vi "RW_LiveVIew.vi"(9 "Task":enum16{"Read", "Write", "Init"}(ring), 11 "Plots":refnum<vi>[](array[refnum])) -> ()   [LabVIEW 2022 SP3]
uses:
  <vilib>/Utility/miscctls.llb/LVRangeTypeDef.ctl
panel:
  out "Data":T1[][](array[typedef])
  out "Pref Path":path
  out "File Out":string
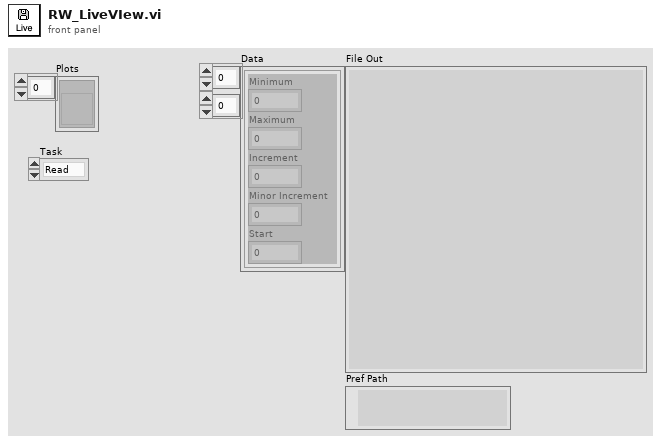
[diagram p1: front panel]
types:
  T1 = typedef "LVRangeTypeDef.ctl" = cluster{"Minimum":dbl, "Maximum":dbl, "Increment":dbl, "Minor Increment":dbl, "Start":dbl}
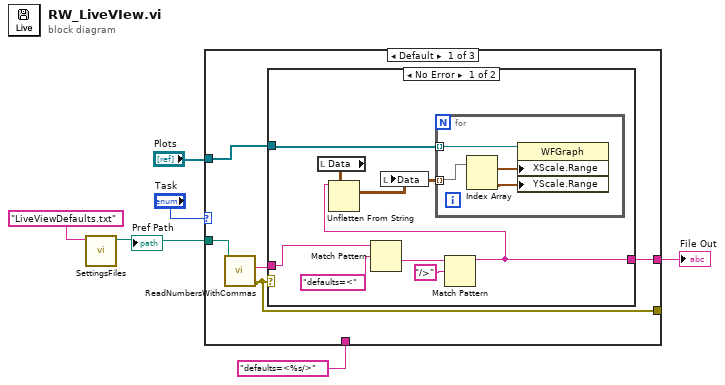
[diagram p0: block diagram]
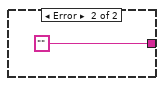
[diagram p2: hidden frame]
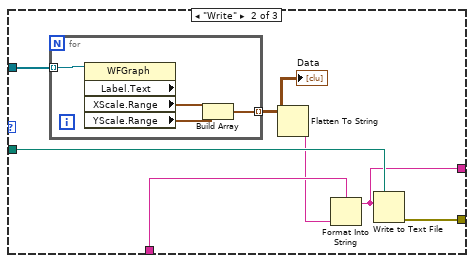
[diagram p3: hidden frame]
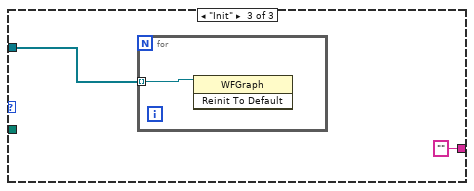
[diagram p4: hidden frame]
diagram:
  n1 = call "SettingsFiles.vi"("settings file name"="LiveViewDefaults.txt" ("name or relative path")) -> ("file path"=w1:path)  [unwired: 9 in, 1 out]
  "Pref Path" <- w1
  n2 = case shown="Default" "Task" {
    tunnel: w1 -> [w11 w31 _]
    tunnel: [w9 w30 _] -> _
    tunnel: [w8 w25 "" ("Notes")] -> w6
    tunnel: "defaults=<%s/>" ("format string") -> [_ w29 _]
    tunnel: "Plots" -> [w7 w28 w37]
    frame Default {
      n3 = call "ReadNumbersWithCommas.vi"("file (use dialog)"=w11) -> ("error out"=w9:errorcluster, "text"=w10:string)  [unwired: 7 in, 2 out]
      n4 = case shown="No Error" w9 {
        tunnel: [w12 "" ("Notes")] -> w8
        tunnel: w10 -> [w19 _]
        tunnel: w7 -> [w14 _]
        frame No Error {
          n5 = local read "Data"() -> (w15:T1[][])
          n6 = Match Pattern(string=w19, regular expression="defaults=<" ("format string")) -> (after substring=w18:string)  [unwired: 1 in, 3 out]
          n7 = Match Pattern(string=w18, regular expression="/>" ("format string")) -> (before substring=w12:string)  [unwired: 1 in, 3 out]
          n8 = Unflatten From String(type=w15, binary string=w12) -> (value=w13:T1[][])  [unwired: 3 in, 2 out]
          n9 = local write "Data"(w13) -> ()
          n10 = for {
            tunnel: w14 -> [w23] mode=indexing
            tunnel: w13 -> [w22] mode=indexing
            n11 = Index Array(array=w22) -> (element #1=w21:T1, element #2=w20:T1)  [unwired: 2 in]
            n12 = property on="Property Node" class="WFGraph"(reference=w23, "XScale.Range"=w21, "YScale.Range"=w20) -> ()  [unwired: 1 in, 2 out]
          }
        }
        frame Error {
        }
      }
    }
    frame "Write" {
      n13 = for {
        tunnel: w28 -> [w35] mode=indexing
        tunnel: [w32] -> w27 mode=indexing
        n14 = property on="Property Node" class="WFGraph" props=["Label", "Text", "XScale", "Range", "YScale", "Range"](reference=w35) -> ("XScale.Range"=w34:T1, "YScale.Range"=w33:T1)  [unwired: 1 in, 3 out]
        n15 = Build Array(w34, w33) -> (w32:T1[])
      }
      "Data" <- w27
      n16 = Flatten To String(anything=w27) -> (data string=w26:string)  [unwired: 3 in, 2 out]
      n17 = Format Into String(format string=w29, w26) -> (resulting string=w25:string)  [unwired: 2 in, 1 out]
      n18 = Write to Text File(file (use dialog)=w31, text=w25) -> (error out=w30:errorcluster)  [unwired: 2 in, 2 out]
    }
    frame "Init" {
      n19 = for {
        tunnel: w37 -> [w38] mode=indexing
        n20 = invoke on="Invoke Node" class="WFGraph" method="Reinit To Default"(reference=w38) -> ()  [unwired: 2 in, 3 out]
      }
    }
  }
  "File Out" <- w6
